vi "FindLinePolygonIntersectionFaces.vi"(2 "Polygon":T1, 3 "ExitPoint":T2, 4 "EntryPoint":T2) -> (0 "Exit Face":i32, 1 "Entry Face":i32)   [LabVIEW 2017, in "ArgosLib.lvlib"]
uses:
  ArgosLib.lvlib
  TypeDefs/Point2D.ctl
  TypeDefs/Polygon2D.ctl
panel:
  out "ClosestExitDist":dbl format="%#_13g"
  out "ClosestEntryDist":dbl format="%#_13g"
  # "Entry Face is index of point at end of polygon\nedge nearest the specified entry point"
  # "Exit Face is index of point at end of polygon\nedge nearest the specified exit point"
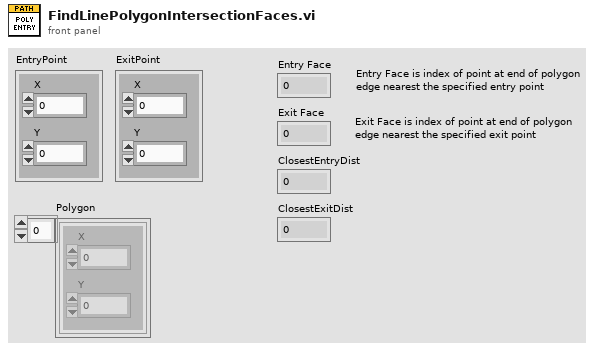
[diagram p1: front panel]
types:
  T1 = typedef "ArgosLib.lvlib/Polygon2D.ctl" = T2[]
  T2 = typedef "ArgosLib.lvlib/Point2D.ctl" = cluster{"X":dbl, "Y":dbl}
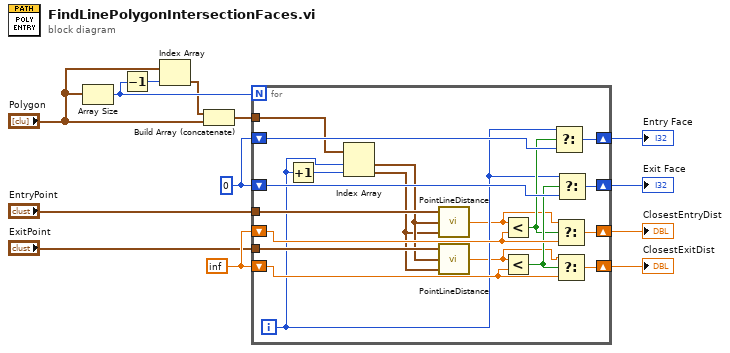
[diagram p0: block diagram]
diagram:
  w8 = 0
  w12 = inf
  n1 = Array Size(array="Polygon") -> (size(s)=w4:i32)
  n2 = Decrement(x=w4) -> (x-1=w5:i32)
  n3 = Index Array(array="Polygon", index=w5) -> (element=w3:T2)
  n4 = Build Array (concatenate)(w3, "Polygon") -> (w1:T1)
  n5 = for {
    N: w4 -> [_]
    shift-right: [w32] -> w13
    shift-left: w12 -> [w31]
    shift-right: [w28] -> w11
    shift-left: w12 -> [w27]
    shift-right: [w30] -> w10
    shift-left: w8 -> [w29]
    shift-right: [w26] -> w9
    shift-left: w8 -> [w25]
    tunnel: "EntryPoint" -> [w22]
    tunnel: "ExitPoint" -> [w21]
    tunnel: w1 -> [w20]
    i -> [w19]
    n6 = Increment(x=w19) -> (x+1=w18:i32)
    n7 = Index Array(array=w20, index #1=w19, index #2=w18) -> (element #1=w17:T2, element #2=w16:T2)
    n8 = call "PointLineDistance.vi"("LinePoint2"=w16, "LinePoint1"=w17, "TestPoint"=w22) -> ("Distance"=w15:dbl)
    n9 = call "PointLineDistance.vi"("LinePoint2"=w16, "LinePoint1"=w17, "TestPoint"=w21) -> ("Distance"=w14:dbl)
    n10 = Less?(x=w15, y=w27) -> (x < y?=w23:bool)
    n11 = Less?(x=w14, y=w31) -> (x < y?=w24:bool)
    n12 = Select(t=w19, s=w23, f=w29) -> (s? t:f=w30:i32)
    n13 = Select(t=w15, s=w23, f=w27) -> (s? t:f=w28:dbl)
    n14 = Select(t=w14, s=w24, f=w31) -> (s? t:f=w32:dbl)
    n15 = Select(t=w19, s=w24, f=w25) -> (s? t:f=w26:i32)
  }
  "Entry Face" <- w10
  "Exit Face" <- w9
  "ClosestEntryDist" <- w11
  "ClosestExitDist" <- w13
